vi "Copy.vi"(7 "Copy Enabled?":bool, 8 "error in (no error)":errorcluster, 11 "Test Configs In":T1) -> (0 "error out":errorcluster, 3 "Test Configs Out":T1)   [LabVIEW 2015]
doc: "Latch the active array element for copy"
uses:
  Type Defs/Sequence Parameters Ref.ctl
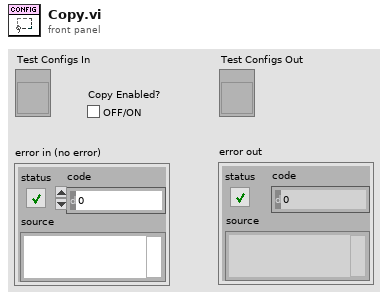
[diagram p1: front panel]
types:
  T1 = typedef "Sequence Parameters Ref.ctl" = refnum<vi>
  T2 = typedef "Sequence Parameters.ctl" = cluster{"Test Name":string, "Target":T3, "Host IP Address":string, "Target IP Address":string, "Shared Variable Host":enum16{"Target", "Host"}, "Shared Variable Writer":enum16{"Target", "Host"}, "Variable Data Type":T4, "# of Variables per Library":u16, "Update Rate (Hz)":dbl, "Read Rate (Hz)":dbl, "Floor":u32, "Ceiling":u32, "Delta":u32}
  T3 = typedef "Target Type.ctl" = enum16{"cRIO-9012", "cRIO-9014", "cRIO-9022", "cRIO-9023", "cRIO-9024", "cRIO-9025", "cRIO-9068", "cRIO-9073", "cRIO-9074", "cRIO-9075", "cRIO-9076", "cRIO-9081", "cRIO-9082", "myRIO-1900", "myRIO-1950", "PXI-8101", "PXI-8115", "PXI-8119", "PXI-8820", "PXIe-8100", "PXIe-8101", "PXIe-8133", "PXIe-8135", "PXIe-8820", "sbRIO-9605", "sbRIO-9606", "sbRIO-9623", "sbRIO-9626", "sbRIO-9633", "sbRIO-9636", "Unlisted (Linux-RT)", "Unlisted (PharLap)", "Unlisted (VxWorks)", "Windows Target"}
  T4 = typedef "Variable Data Type.ctl" = enum16{"U8", "U16", "U32", "U64", "I8", "I16", "I32", "I64", "Single", "Double", "Boolean", "String"}
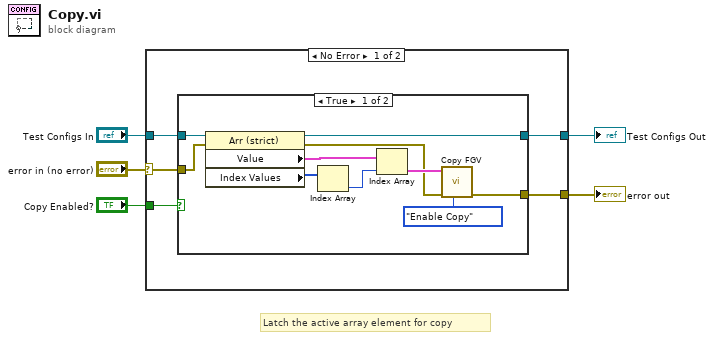
[diagram p0: block diagram]
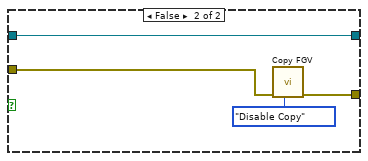
[diagram p2: hidden frame]
diagram:
  # "Latch the active array element for copy"
  n1 = case shown="No Error" "error in (no error)" {
    selector: "error in (no error)" -> [w9 w25]
    tunnel: "Test Configs In" -> [w10 w26]
    tunnel: [w8 w26] -> w2
    tunnel: [w6 w25] -> w3
    tunnel: "Copy Enabled?" -> [w7 _]
    frame No Error {
      n2 = case shown="True" w7 {
        tunnel: w10 -> [w20 w22]
        tunnel: w9 -> [w19 w21]
        tunnel: [w12 w22] -> w8
        tunnel: [w11 w23] -> w6
        frame True {
          n3 = property class="Arr (strict)"(reference=w20, error in=w19) -> (reference out=w12:T1, error out=w14:errorcluster, "Value"=w17:T2[], "Index Values"=w18:u32[])
          n4 = Index Array(array=w18) -> (element=w16:u32)  [unwired: 1 in]
          n5 = Index Array(array=w17, index=w16) -> (element=w15:T2)
          n6 = call "Copy FGV.vi"("Mode"=enum16{"Enable Copy", "Disable Copy", "Read"}."Enable Copy", "error in (no error)"=w14, "Element to Write"=w15) -> ("error out"=w11:errorcluster)  [unwired: 6 in, 2 out]
        }
        frame False {
          n7 = call "Copy FGV.vi"("Mode"=enum16{"Enable Copy", "Disable Copy", "Read"}."Disable Copy", "error in (no error)"=w21) -> ("error out"=w23:errorcluster)  [unwired: 7 in, 2 out]
        }
      }
    }
    frame Error {
    }
  }
  "Test Configs Out" <- w2
  "error out" <- w3
